vi "Read Method Results.vi"(11 "Test Case Result In":refnum<class "Test Case Result.lvclass">) -> (2 "Method Results":T1(c390), 3 "Test Case Result Out":refnum<class "Test Case Result.lvclass">)   [LabVIEW 2020, in "Test Case Result.lvclass"]
uses:
  Test Case Result.lvclass
  Method Result/Method Result.lvclass
  Test Case Result.lvclass/Test Case Result.ctl
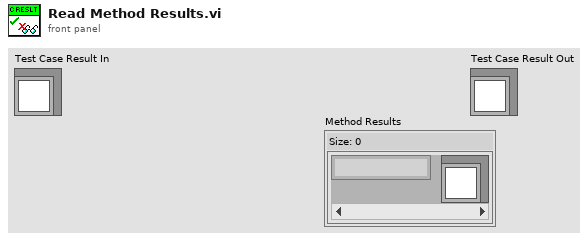
[diagram p1: front panel]
types:
  T1 = map{string, refnum<class "Method Result.lvclass">}
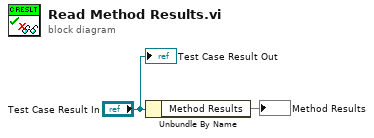
[diagram p0: block diagram]
diagram:
  n1 = Unbundle By Name("Test Case Result In") -> ("Method Results"=→"Method Results":T1)
  "Test Case Result Out" <- "Test Case Result In"
